vi "test q.vi"() -> ()   [LabVIEW 2014]
panel:
  in  "Boolean":bool
  out "error out":errorcluster
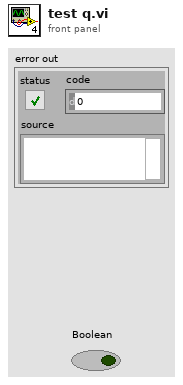
[diagram p1: front panel]
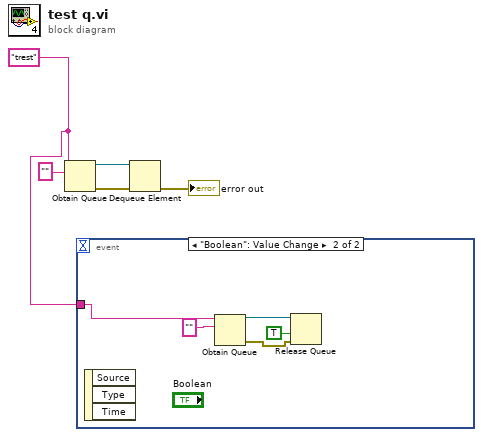
[diagram p0: block diagram]
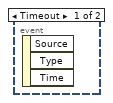
[diagram p2: hidden frame]
diagram:
  w1 = "trest" ("name (unnamed)")
  n1 = Obtain Queue(name (unnamed)=w1, element data type="") -> (queue out=w4:refnum<queue>, error out=w3:errorcluster)  [unwired: 3 in, 1 out]
  n2 = event shown="[1] \"Boolean\": Value Change" {
    selector: _ -> [_ _]
    dyn-events: _ -> [_ _]
    timeout: _ -> [_ _]
    tunnel: w1 -> [_ w10]
    event Timeout {
      n3 = event-data() -> ()  [unwired: 1 in, 3 out]
    }
    event "Boolean": Value Change {
      n4 = event-data() -> ()  [unwired: 1 in, 3 out]
      n5 = Obtain Queue(name (unnamed)=w10, element data type="") -> (queue out=w9:refnum<queue>, error out=w7:errorcluster)  [unwired: 3 in, 1 out]
      n6 = Release Queue(queue=w9, force destroy? (F)=TRUE, error in (no error)=w7) -> ()  [unwired: 3 out]
    }
  }
  n7 = Dequeue Element(queue=w4, error in (no error)=w3) -> (error out=→"error out":errorcluster)  [unwired: 1 in, 3 out]
